vi "visionDirection.vi"(8 "Error In":errorcluster) -> (0 "Error Out":errorcluster, 3 "Direction":string)   [LabVIEW 2019]
uses:
  WSCbot_V3_Toolkit.lvlibp
panel:
  out "left | right?":bool
  out "success?":bool
  in  "Stop Button":bool
  out "Score":sgl
  out "Original":T1(plugin-control)
  out "Image Out":T1(plugin-control)
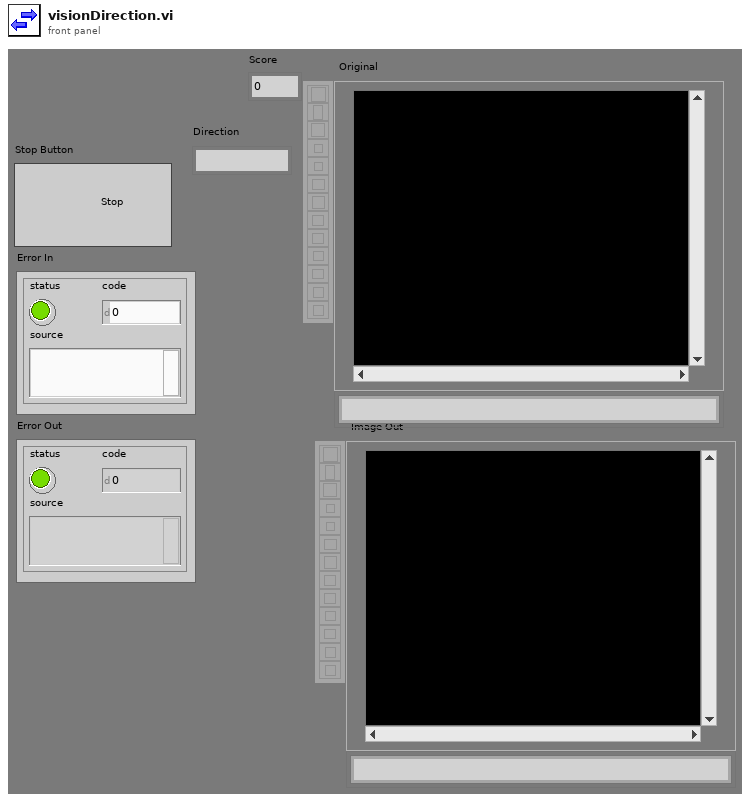
[diagram p1: front panel]
types:
  T1 = typedef "IMAQ Image.ctl" = refnum<image>
  T2 = typedef "IMAQ GM Match Report.ctl" = cluster{"Position":cluster{"x":sgl, "y":sgl}, "Angle":sgl, "Scale":sgl, "Score":sgl, "Bounding Box":cluster{"x":sgl, "y":sgl}[], "Contrast Reversed":bool, "Occlusion %":sgl, "Template Target Curve Score":sgl, "Target Template Curve Score":sgl, "Correlation Score":sgl}
  T3 = cluster{"Matches (Pattern Matching 1)[0]":T2, "Matches (Pattern Matching 1)[1]":T2, "Matches (Pattern Matching 1)[2]":T2, "Matches (Pattern Matching 1)[3]":T2, "Matches (Pattern Matching 1)[4]":T2, "Matches (Pattern Matching 1)[5]":T2, "Matches (Pattern Matching 1)[6]":T2, "Matches (Pattern Matching 1)[7]":T2, "Matches (Pattern Matching 1)[8]":T2}
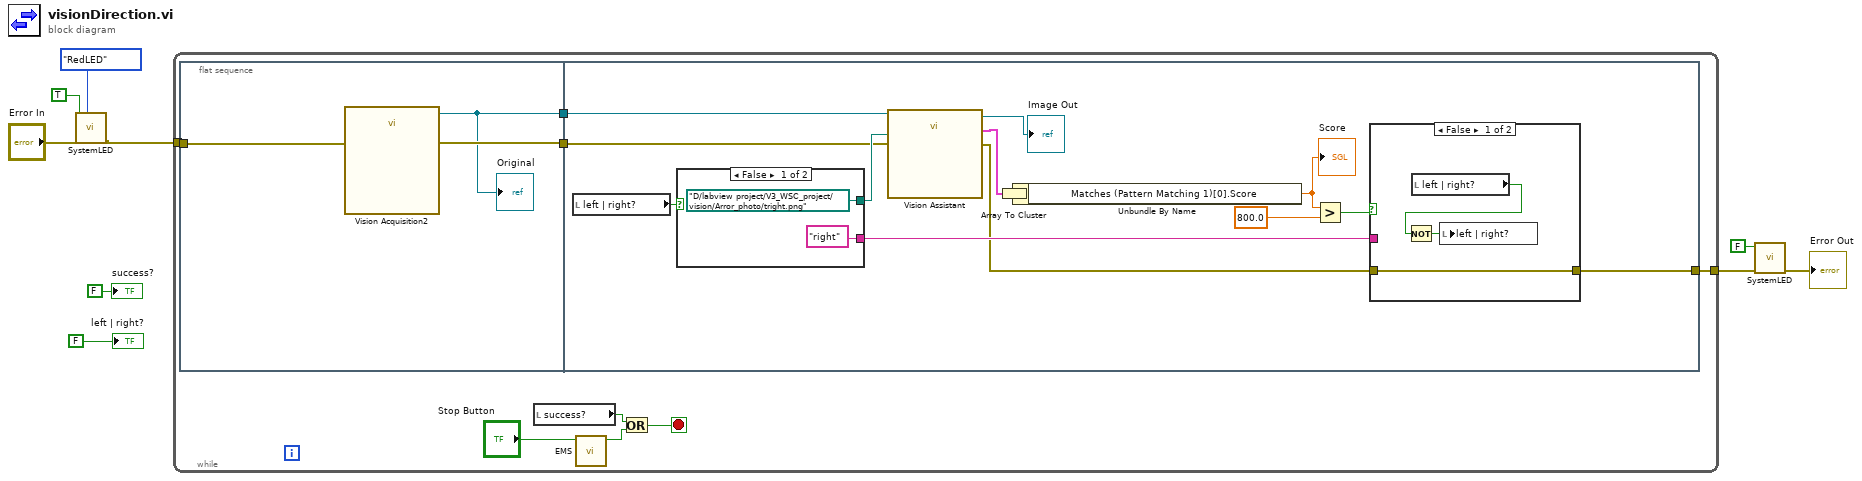
[diagram p0: block diagram]
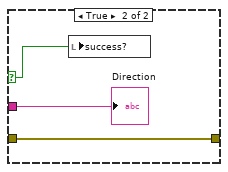
[diagram p2: hidden frame]
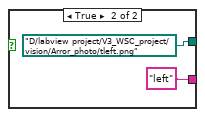
[diagram p3: hidden frame]
diagram:
  n1 = call "SystemLED.vi"("SelectColor"=enum16{"RedLED", "GreenLED", "YellowLED"}."RedLED", "error in"="Error In", "Set"=TRUE) -> ("error out"=w5:errorcluster)  [unwired: 8 in]
  n2 = while {
    tunnel: w5 -> [w17]
    tunnel: [w16] -> w2
    stop <- w12 stop-if-true
    n3 = flat-sequence {
      tunnel: w17 -> [w20]
      tunnel: [w19] -> w15
      tunnel: [w18] -> w14
      tunnel: [w30] -> w16
      tunnel: w15 -> [w23]
      tunnel: w14 -> [w22]
      frame #0 {
        n4 = call "Vision Acquisition2"("error in"=w20) -> ("Image Out"=w18:T1, "error out"=w19:errorcluster)  [unwired: 25 in]
        "Original" <- w18
      }
      frame #1 {
        n5 = local read "left | right?"() -> (w21:bool)
        n6 = case shown="False" w21 {
          tunnel: ["right" "left"] -> w28
          tunnel: [path "D:/labview project/V3_WSC_project/vision/Arror_photo/tright.png" ("Template File Path (Pattern Matching 1)") path "D:/labview project/V3_WSC_project/vision/Arror_photo/tleft.png" ("Template File Path (Pattern Matching 1)")] -> w24
          frame False {
          }
          frame True {
          }
        }
        n7 = call "Vision Assistant"("Image In"=w22, "Template File Path (Pattern Matching 1)"=w24, "error in"=w23) -> ("Image Out"=→"Image Out":T1, "Matches (Pattern Matching 1)"=w26:T2[], "error out"=w27:errorcluster)  [unwired: 22 in]
        n8 = Array To Cluster(array=w26) -> (cluster=w33:T3)
        n9 = Unbundle By Name(w33) -> ("Matches (Pattern Matching 1)[0].Score"=w31:sgl)
        "Score" <- w31
        n10 = Greater?(x=w31, y=sgl 800.0) -> (0:w29:bool)
        n11 = case shown="False" w29 {
          selector: w29 -> [_ w37]
          tunnel: w27 -> [w36 w39]
          tunnel: [w36 w39] -> w30
          tunnel: w28 -> [_ w38]
          frame False {
            n12 = local read "left | right?"() -> (w35:bool)
            n13 = Not(x=w35) -> (.not. x?=w34:bool)
            n14 = local write "left | right?"(w34) -> ()
          }
          frame True {
            n15 = local write "success?"(w37) -> ()
            "Direction" <- w38
          }
        }
      }
    }
    n16 = local read "success?"() -> (w13:bool)
    n17 = call "EMS.vi"("ProgramStop"="Stop Button") -> ("EMS"=w11:bool)  [unwired: 9 in, 1 out]
    n18 = Or(x=w13, y=w11) -> (x .or. y?=w12:bool)
  }
  n19 = call "SystemLED.vi"("error in"=w2, "Set"=FALSE) -> ("error out"=→"Error Out":errorcluster)  [unwired: 9 in]
  "success?" <- FALSE ("success?")
  "left | right?" <- FALSE ("left | right?")
